vi "close.vi"(0 "连接ID":refnum<k5>) -> ()   [LabVIEW 2017]
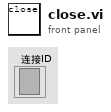
[diagram p1: front panel]
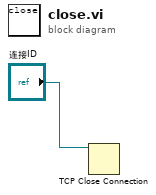
[diagram p0: block diagram]
diagram:
  n1 = TCP Close Connection(connection ID="连接ID") -> ()  [unwired: 2 in, 2 out]
